vi "Annotate Frame.vi"(6 "Codec":string, 7 "Clip width":i32, 8 "error in (no error)":errorcluster, 9 "Annotation Type":T11, 10 "Annotation":string, 11 "Frame Grabber Data In in":T1={"Camera Session"="", "Frame"=refnum, "AVI Refnum"=refnum, "Codecs"=[], "Frame number"=0, "Tracking File Refnum"=refnum, "Tick Count"=0, "Probe Object"=refnum, "Playback Probe Data"=[], "Rigid Body"={"Position"={"x (mm)"=0.0, "y (mm)"=0.0, "z (mm)"=0.0}, "Orientation"={"Pitch (rad)"=0.0, "Yaw (rad)"=0.0, "Roll (rad)"=0.0}, "Quaternion"={"qx"=0.0, "qy"=0.0, "qz"=0.0, "qw"=0.0}, "Tracked?"=FALSE}, "Total no frames playback"=0, "Video FPS"=0.0, "Camera connected?"=FALSE, "Scene"=refnum, "Cropped Frame"=refnum, "Tracker FPS"=0.0, "Crop ROI"=[], "Presentation Values"=[], "Elapsed time (ms)"=0, "Camera frames playback"=0, "Refnums"={"Live Refnum"=refnum, "Record Refnum"=refnum, "Playback Refnum"=refnum, "Frame Slider Refnum"=refnum, "Pause Refnum"=refnum, "Home Refnum"=refnum, "Set Crop Refnum"=refnum, "Clear Crop Refnum"=refnum, "stop refnum"=refnum, "Playback Rate Refnum"=refnum, "Presentation Refnum"=refnum, "Crop Time Frame Slider Refnum"=refnum, "Cancel Save Refnum"=refnum, "Reverse Playback Refnum"=refnum, "Recording Settings Refnum"=refnum, "Continuous Playback Refnum"=refnum, "Annotation Refnum"=refnum, "Export All Refnum"=refnum, "Export List Refnum"=refnum, "Fill List Refnum"=refnum, "Save Crop Refnum"=refnum, "Skip Forward Refnum"=refnum, "Skip Backward Refnum"=refnum, "Single Annotation Refnum"=refnum, "Load Refnum"=refnum, "Set Start Refnum"=refnum, "Set End Refnum"=refnum, "Add to List Refnum"=refnum, "List of Annotations Refnum"=refnum, "Camera Frame Refnum"=refnum}, "Dimensions"={"Probe Dimensions"={"Probe Width"=0.0, "Probe Depth"=1.0, "Probe Height"=0.0}, "Room Dimensions"={"Room Width"=0.0, "Room Depth"=0.0, "Room Height"=0.0}}, "Playback Data As Strings"=[], "Cropped Tracking File Refnum"=refnum, "Cropped AVI Refnum"=refnum, "Header"=[], "Total euclidian distance"=0.0, "Annotation File Path"=path "", "Playback File Path"=path "", "Size per frame"=0.0, "Ground Truth File Refnum"=refnum, "Annotation Array"=[], "Annotation TIFFs Folder"=path "", "overwriting open file?"=FALSE}) -> (0 "error out":errorcluster, 2 "saving?":bool, 3 "Frame Grabber Data Out":T1={"Camera Session"="", "Frame"=refnum, "AVI Refnum"=refnum, "Codecs"=[], "Frame number"=0, "Tracking File Refnum"=refnum, "Tick Count"=0, "Probe Object"=refnum, "Playback Probe Data"=[], "Rigid Body"={"Position"={"x (mm)"=0.0, "y (mm)"=0.0, "z (mm)"=0.0}, "Orientation"={"Pitch (rad)"=0.0, "Yaw (rad)"=0.0, "Roll (rad)"=0.0}, "Quaternion"={"qx"=0.0, "qy"=0.0, "qz"=0.0, "qw"=0.0}, "Tracked?"=FALSE}, "Total no frames playback"=0, "Video FPS"=0.0, "Camera connected?"=FALSE, "Scene"=refnum, "Cropped Frame"=refnum, "Tracker FPS"=0.0, "Crop ROI"=[], "Presentation Values"=[], "Elapsed time (ms)"=0, "Camera frames playback"=0, "Refnums"={"Live Refnum"=refnum, "Record Refnum"=refnum, "Playback Refnum"=refnum, "Frame Slider Refnum"=refnum, "Pause Refnum"=refnum, "Home Refnum"=refnum, "Set Crop Refnum"=refnum, "Clear Crop Refnum"=refnum, "stop refnum"=refnum, "Playback Rate Refnum"=refnum, "Presentation Refnum"=refnum, "Crop Time Frame Slider Refnum"=refnum, "Cancel Save Refnum"=refnum, "Reverse Playback Refnum"=refnum, "Recording Settings Refnum"=refnum, "Continuous Playback Refnum"=refnum, "Annotation Refnum"=refnum, "Export All Refnum"=refnum, "Export List Refnum"=refnum, "Fill List Refnum"=refnum, "Save Crop Refnum"=refnum, "Skip Forward Refnum"=refnum, "Skip Backward Refnum"=refnum, "Single Annotation Refnum"=refnum, "Load Refnum"=refnum, "Set Start Refnum"=refnum, "Set End Refnum"=refnum, "Add to List Refnum"=refnum, "List of Annotations Refnum"=refnum, "Camera Frame Refnum"=refnum}, "Dimensions"={"Probe Dimensions"={"Probe Width"=0.0, "Probe Depth"=1.0, "Probe Height"=0.0}, "Room Dimensions"={"Room Width"=0.0, "Room Depth"=0.0, "Room Height"=0.0}}, "Playback Data As Strings"=[], "Cropped Tracking File Refnum"=refnum, "Cropped AVI Refnum"=refnum, "Header"=[], "Total euclidian distance"=0.0, "Annotation File Path"=path "", "Playback File Path"=path "", "Size per frame"=0.0, "Ground Truth File Refnum"=refnum, "Annotation Array"=[], "Annotation TIFFs Folder"=path "", "overwriting open file?"=FALSE})   [LabVIEW 2017]
uses:
  Controls/Frame Grabber Data.ctl
  <vilib>/userdefined/High Color/IMAQdx.ctl
  <vilib>/vision/Image Controls.llb/IMAQ Image.ctl
  <vilib>/vision/Avi.llb/IMAQ AVI2 Refnum.ctl
  Controls/Rigid Body Info.ctl
  Controls/Position.ctl
  Controls/Orientation.ctl
  Controls/Refnums.ctl
  Controls/Recording Settings.ctl
  Controls/Operator Settings.ctl
  Controls/Operator.ctl
  Controls/Patient Settings.ctl
  Controls/Dimensions.ctl
  Controls/Room Dimensions.ctl
  Controls/Annotation Type.ctl
  <vilib>/Utility/file.llb/Read Delimited Spreadsheet (string).vi
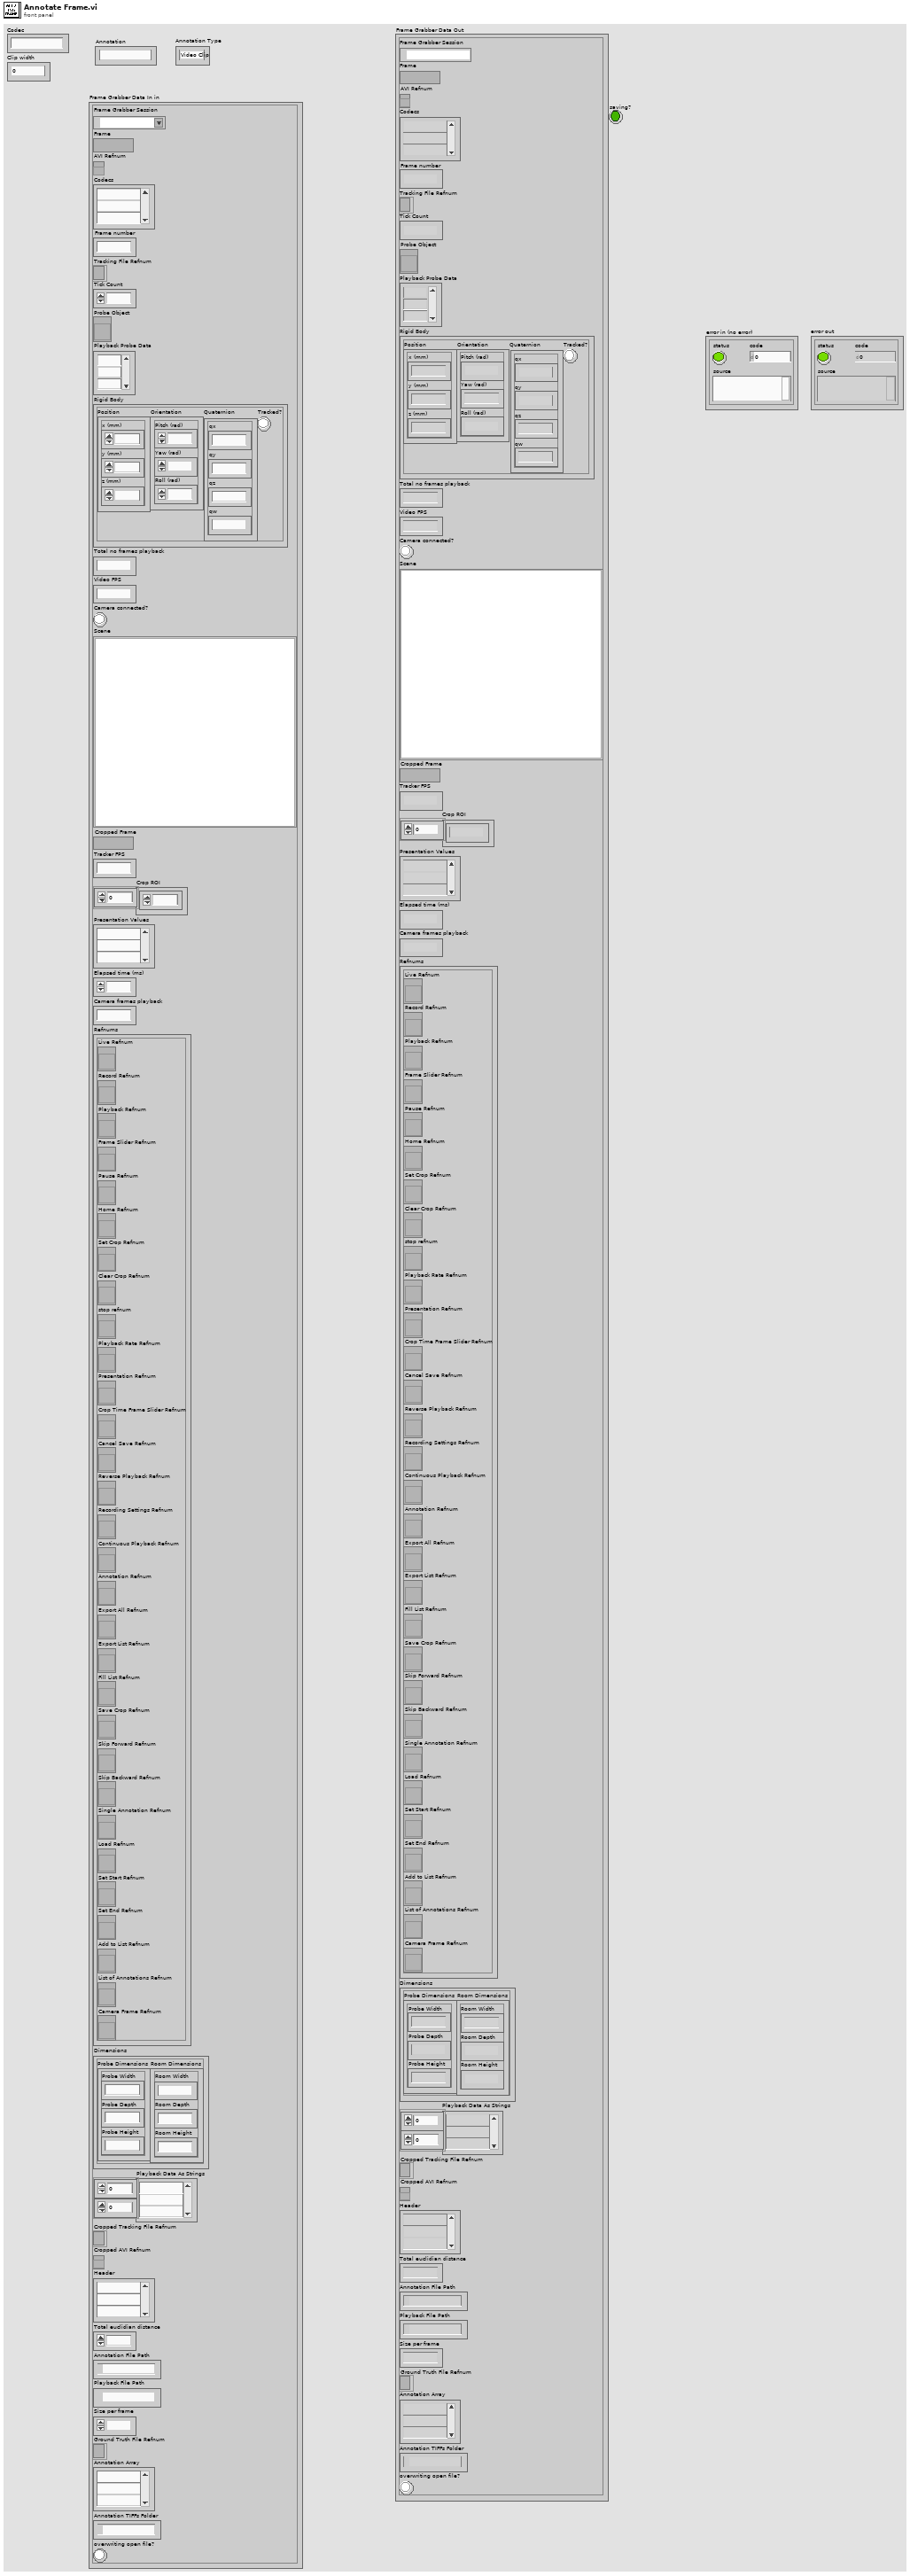
[diagram p1: front panel]
types:
  T1 = typedef "Frame Grabber Data.ctl" = cluster{"Camera Session":T2, "Frame":T3, "AVI Refnum":T4, "Codecs":string[], "Frame number":u32, "Tracking File Refnum":refnum<file>, "Tick Count":u32, "Probe Object":refnum<vi>, "Playback Probe Data":dbl[][], "Rigid Body":T5, "Total no frames playback":i32, "Video FPS":dbl, "Camera connected?":bool, "Scene":refnum<vi>, "Cropped Frame":T3, "Tracker FPS":dbl, "Crop ROI":i32[], "Presentation Values":string[], "Elapsed time (ms)":u32, "Camera frames playback":u32, "Refnums":T8, "Dimensions":T9, "Playback Data As Strings":string[][], "Cropped Tracking File Refnum":refnum<file>, "Cropped AVI Refnum":T4, "Header":string[], "Total euclidian distance":dbl, "Annotation File Path":path, "Playback File Path":path, "Size per frame":dbl, "Ground Truth File Refnum":refnum<file>, "Annotation Array":string[], "Annotation TIFFs Folder":path, "overwriting open file?":bool}
  T2 = typedef "IMAQdx.ctl" = refnum<k21>
  T3 = typedef "IMAQ Image.ctl" = refnum<image>
  T4 = typedef "IMAQ AVI2 Refnum.ctl" = refnum<k20>
  T5 = typedef "Rigid Body Info.ctl" = cluster{"Position":T6, "Orientation":T7, "Quaternion":cluster{"qx":sgl, "qy":sgl, "qz":sgl, "qw":sgl}, "Tracked?":bool}
  T6 = typedef "Position.ctl" = cluster{"x (mm)":sgl, "y (mm)":sgl, "z (mm)":sgl}
  T7 = typedef "Orientation.ctl" = cluster{"Pitch (rad)":sgl, "Yaw (rad)":sgl, "Roll (rad)":sgl}
  T8 = typedef "Refnums.ctl" = cluster{"Live Refnum":refnum<vi>, "Record Refnum":refnum<vi>, "Playback Refnum":refnum<vi>, "Frame Slider Refnum":refnum<vi>, "Pause Refnum":refnum<vi>, "Home Refnum":refnum<vi>, "Set Crop Refnum":refnum<vi>, "Clear Crop Refnum":refnum<vi>, "stop refnum":refnum<vi>, "Playback Rate Refnum":refnum<vi>, "Presentation Refnum":refnum<vi>, "Crop Time Frame Slider Refnum":refnum<vi>, "Cancel Save Refnum":refnum<vi>, "Reverse Playback Refnum":refnum<vi>, "Recording Settings Refnum":refnum<vi>, "Continuous Playback Refnum":refnum<vi>, "Annotation Refnum":refnum<vi>, "Export All Refnum":refnum<vi>, "Export List Refnum":refnum<vi>, "Fill List Refnum":refnum<vi>, "Save Crop Refnum":refnum<vi>, "Skip Forward Refnum":refnum<vi>, "Skip Backward Refnum":refnum<vi>, "Single Annotation Refnum":refnum<vi>, "Load Refnum":refnum<vi>, "Set Start Refnum":refnum<vi>, "Set End Refnum":refnum<vi>, "Add to List Refnum":refnum<vi>, "List of Annotations Refnum":refnum<vi>, "Camera Frame Refnum":refnum<vi>}
  T9 = typedef "Dimensions.ctl" = cluster{"Probe Dimensions":cluster{"Probe Width":sgl, "Probe Depth":sgl, "Probe Height":sgl}, "Room Dimensions":T10}
  T10 = typedef "Room Dimensions.ctl" = cluster{"Room Width":dbl, "Room Depth":dbl, "Room Height":dbl}
  T11 = typedef "Annotation Type.ctl" = enum16{"Video Clip", "Image"}
  T12 = enum16{"open", "replace", "create", "open or create", "replace or create", "replace or create with confirmation"}
  T13 = cluster{"Width":u32, "Height":u32, "Frames Per Second":u32, "Codec":string, "Has Data":bool}
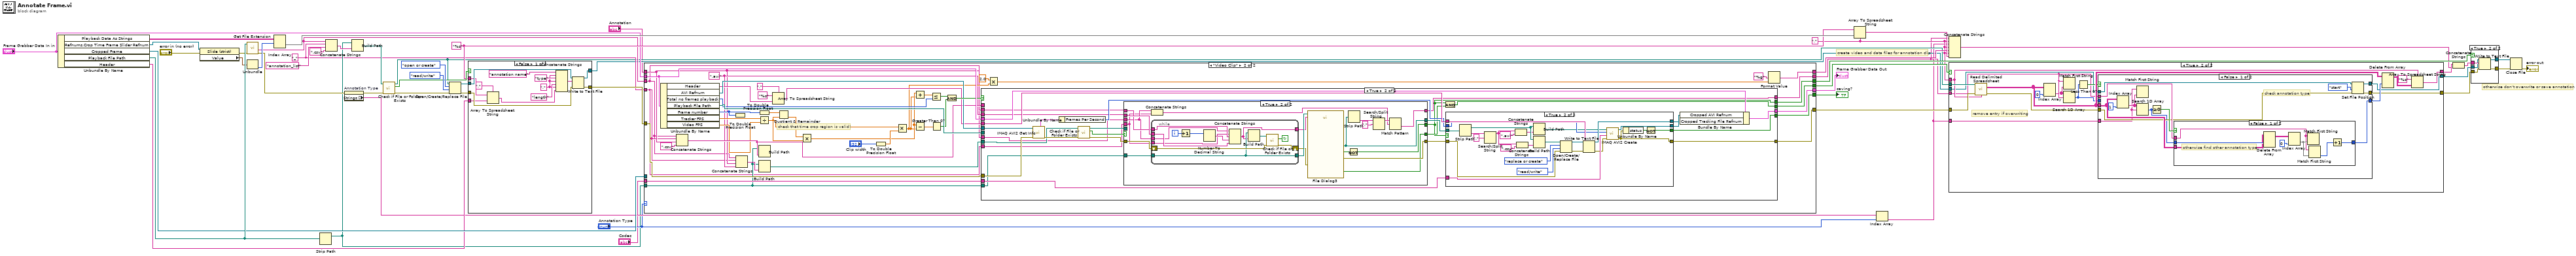
[diagram p0: block diagram]
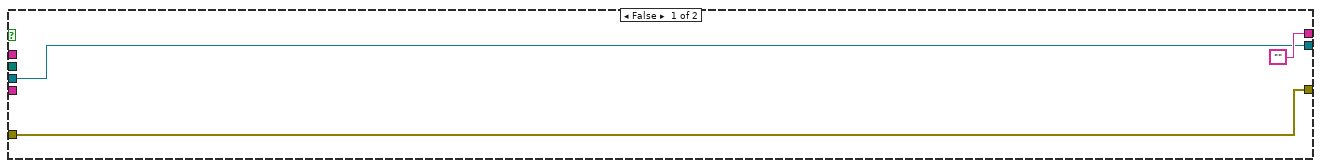
[diagram p2: hidden frame]
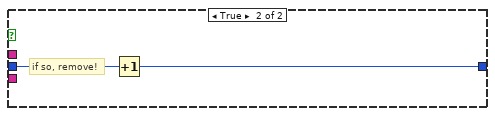
[diagram p3: hidden frame]
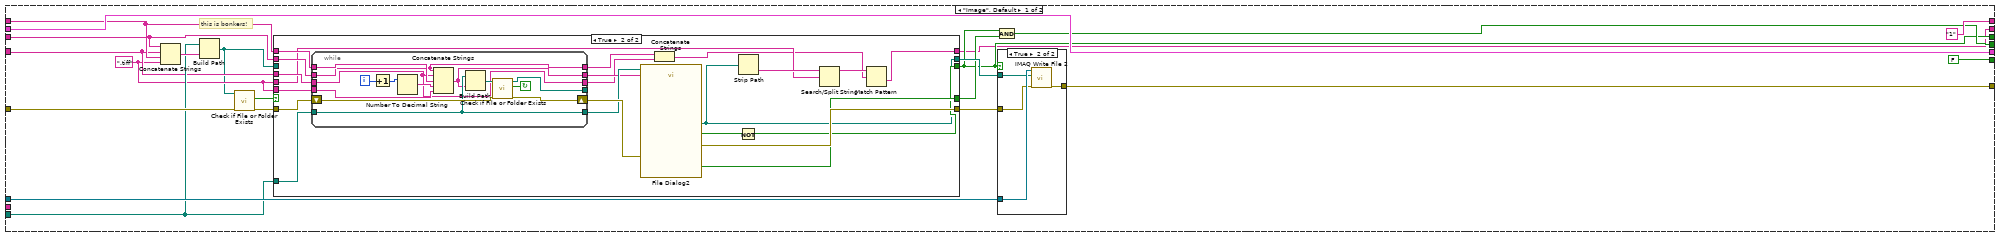
[diagram p6: hidden frame]
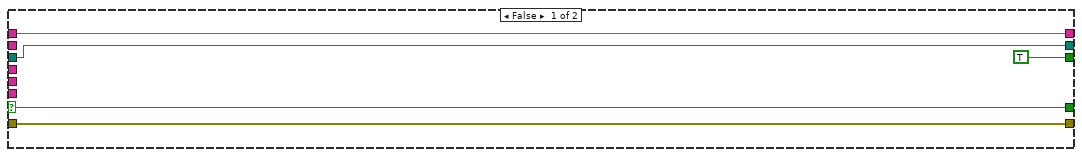
[diagram p7: hidden frame]
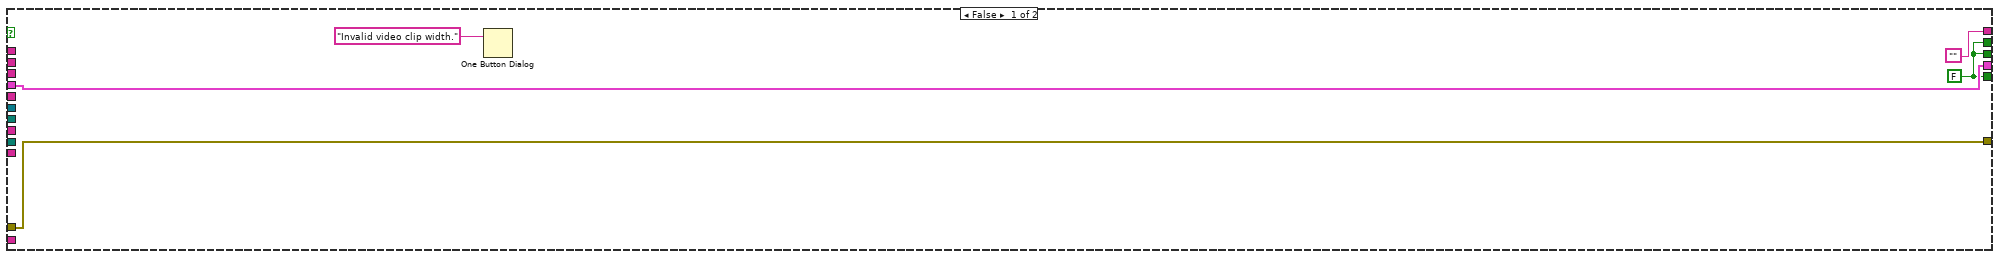
[diagram p9: hidden frame]
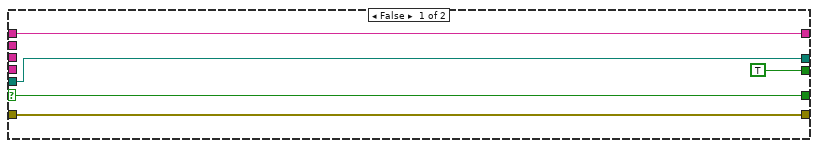
[diagram p10: hidden frame]
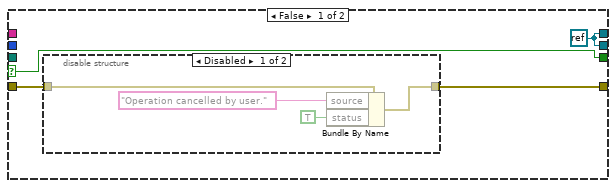
[diagram p11: hidden frame]
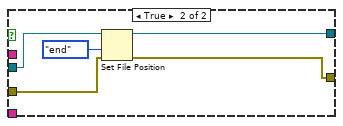
[diagram p13: hidden frame]
diagram:
  w19 = "_" ("string")
  w6 = "," ("delimiter (Tab)")
  w33 = "%s" ("format string")
  # "otherwise don't overwrite or save annotation"
  # "create video and data files for annotation clip"
  n1 = Unbundle By Name("Frame Grabber Data In in") -> ("Playback Data As Strings"=w52:string[][], "Refnums.Crop Time Frame Slider Refnum"=w32:refnum<vi>, "Cropped Frame"=w42:T3, "Playback File Path"=w51:path, "Header"=w39:string[])
  n2 = property class="Slide (strict)"(reference=w32, error in="error in (no error)") -> (error out=w28:errorcluster, "Value"=w31:cluster{i32, i32, i32})  [unwired: 1 out]
  n3 = call <vilib>:"Get File Extension.vi"("error in (no error)"=w28, "file"=w51) -> ("error out"=w27:errorcluster, "filename without extension"=w20:string)  [unwired: 5 in, 3 out]
  n4 = Unbundle(w31) -> (w30:i32)  [unwired: 2 out]
  n5 = Index Array(array=w52, index (row)=w30) -> (element=w34:string[])  [unwired: 1 in]
  n6 = Strip Path(path=w51) -> (stripped path=w21:path)  [unwired: 1 out]
  n7 = Concatenate Strings(w20, w19, "annotation_list" ("string"), ".csv" ("string")) -> (w50:string)
  n8 = property on="Annotation Type" class="Enum (strict)"(error in=w27) -> (error out=w26:errorcluster, "Strings []"=w25:string[])  [unwired: 1 in, 1 out]
  n9 = Build Path(base path=w21, name or relative path=w50) -> (appended path=w41:path)
  n10 = call <vilib>:"Check if File or Folder Exists.vi"("error in (no error)"=w26, "path"=w41) -> ("error out"=w40:errorcluster, "file or folder exists?"=w37:bool, "dup path"=w12:path)  [unwired: 7 in]
  n11 = Open/Create/Replace File(file path (use dialog)=w12, error in=w40, operation (0:open)=T12."open or create", access (0:read/write)=enum16{"read/write", "read-only", "write-only"}."read/write") -> (refnum out=w35:refnum<file>, error out=w38:errorcluster)  [unwired: 2 in, 1 out]
  n12 = case shown="False" w37 {
    tunnel: w39 -> [w59 _]
    tunnel: w38 -> [w64 w70]
    tunnel: [w63 w67] -> w36
    tunnel: w35 -> [w62 w69]
    tunnel: [w61 w68] -> w4
    tunnel: w33 -> [w56 _]
    frame False {
      w53 = "," ("string")
      n13 = Array To Spreadsheet String(delimiter (Tab)=",", array=w59, 3:w56) -> (spreadsheet string=w57:string)
      n14 = Concatenate Strings("annotation name" ("string"), w53, "type" ("string"), w53, "length" ("string"), w53, w57) -> (w60:string)
      n15 = Write to Text File(file (use dialog)=w62, text=w60, error in=w64) -> (refnum out=w61:refnum<file>, error out=w63:errorcluster)  [unwired: 1 in, 1 out]
    }
    frame True {
      n16 = Set File Position(refnum=w69, from (0:start)=enum16{"start", "end", "current"}."end", error in=w70) -> (refnum out=w68:refnum<file>, error out=w67:errorcluster)  [unwired: 1 in]
    }
  }
  n17 = case shown="\"Video Clip\"" "Annotation Type" {
    tunnel: [w91 w178] -> w11
    tunnel: w42 -> [w90 _]
    tunnel: w36 -> [w85 w179]
    tunnel: [w89 w176] -> w23
    tunnel: "Frame Grabber Data In in" -> [w89 w177]
    tunnel: w21 -> [w80 w142]
    tunnel: w20 -> [w78 w138]
    tunnel: w19 -> [w79 w139]
    tunnel: "Annotation" -> [w81 w140]
    tunnel: "Codec" -> [_ w175]
    tunnel: [FALSE ("status") w159] -> w17
    tunnel: ["1" ("output string") w145] -> w15
    tunnel: [w74 w144] -> w14
    tunnel: [w86 w143] -> w13
    tunnel: [w72 w137] -> w2
    frame "Image", Default {
      w73 = ".tiff" ("string")
      # "this is bonkers!"
      n18 = Concatenate Strings(w78, w79, w81, w73) -> (w84:string)
      n19 = Build Path(base path=w80, name or relative path=w84) -> (appended path=w71:path)
      n20 = call <vilib>:"Check if File or Folder Exists.vi"("error in (no error)"=w85, "path"=w71) -> ("error out"=w82:errorcluster, "file or folder exists?"=w83:bool)  [unwired: 7 in, 1 out]
      n21 = case shown="True" w83 {
        selector: w83 -> [w94 _]
        tunnel: w82 -> [w96 w117]
        tunnel: [w96 w115] -> w77
        tunnel: w80 -> [_ w110]
        tunnel: [w92 w104] -> w76
        tunnel: [TRUE w112] -> w74
        tunnel: [w94 w114] -> w75
        tunnel: w81 -> [w93 w111]
        tunnel: w73 -> [_ w109]
        tunnel: w79 -> [_ w108]
        tunnel: w78 -> [_ w107]
        tunnel: w73 -> [_ w102]
        tunnel: [w93 w97] -> w72
        tunnel: w71 -> [w92 _]
        frame False {
        }
        frame True {
          n22 = while {
            shift-right: [w130] -> w116
            shift-left: w117 -> [w123]
            tunnel: [w129] -> _
            tunnel: w111 -> [w125]
            tunnel: w110 -> [w121]
            tunnel: w109 -> [w124]
            tunnel: w108 -> [w119]
            tunnel: w107 -> [w118]
            tunnel: [w121] -> w106
            tunnel: [w120] -> w105
            tunnel: [w119] -> w100
            tunnel: [w118] -> w99
            i -> [w128]
            stop <- w131 continue-if-true
            n23 = Increment(x=w128) -> (x+1=w127:i32)
            n24 = Number To Decimal String(number=w127) -> (decimal integer string=w126:string)  [unwired: 1 in]
            n25 = Concatenate Strings(w118, w119, w125, w126, w124) -> (w120:string)
            n26 = Build Path(base path=w121, name or relative path=w120) -> (appended path=w122:path)
            n27 = call <vilib>:"Check if File or Folder Exists.vi"("error in (no error)"=w123, "path"=w122) -> ("error out"=w130:errorcluster, "file or folder exists?"=w131:bool, "dup path"=w129:path)  [unwired: 7 in]
          }
          n28 = call "File Dialog2"("start path"=w106, "default name"=w105, "error in"=w116) -> ("selected path"=w104:path, "exists"=w114:bool, "cancelled"=w113:bool, "error out"=w115:errorcluster)  [unwired: 9 in]
          n29 = Concatenate Strings(w99, w100) -> (w98:string)
          n30 = Not(x=w113) -> (.not. x?=w112:bool)
          n31 = Strip Path(path=w104) -> (name=w103:string)  [unwired: 1 out]
          n32 = Search/Split String(string=w103, search string/char (-)=w102) -> (substring before match=w101:string)  [unwired: 1 in, 2 out]
          n33 = Match Pattern(string=w101, regular expression=w98) -> (after substring=w97:string)  [unwired: 1 in, 3 out]
        }
      }
      n34 = And(x=w74, y=w75) -> (x .and. y?=w86:bool)
      n35 = case shown="True" w74 {
        tunnel: [w132 w133] -> w91
        tunnel: w90 -> [_ w136]
        tunnel: w77 -> [w132 w135]
        tunnel: w76 -> [_ w134]
        frame False {
        }
        frame True {
          n36 = call-poly "IMAQ Write File 2"("error in (no error)"=w135, "File Path"=w134, "Image"=w136) -> ("error out"=w133:errorcluster)  [unwired: 7 in, 1 out]
        }
      }
    }
    frame "Video Clip" {
      w141 = ".avi" ("string")
      # "check that time crop region is valid!"
      n37 = Unbundle By Name(w177) -> ("Header"=w170:string[], "AVI Refnum"=w171:T4, "Total no frames playback"=w161:i32, "Playback File Path"=w174:path, "Frame number"=w154:u32, "Tracker FPS"=w158:dbl, "Video FPS"=w157:dbl)
      n38 = Concatenate Strings(w138, w139, w140, ".csv" ("string")) -> (w164:string)
      n39 = To Double Precision Float(number=w154) -> ()  [unwired: 1 out]
      n40 = Concatenate Strings(w138, w139, w140, w141) -> (w180:string)
      n41 = To Double Precision Float(number=w154) -> (double precision float=w152:dbl)
      n42 = Divide(x=w158, y=w157) -> (x/y=w150:dbl)
      n43 = Build Path(base path=w142, name or relative path=w164) -> ()  [unwired: 1 out]
      n44 = Build Path(base path=w142, name or relative path=w180) -> (appended path=w166:path)
      n45 = Array To Spreadsheet String(delimiter (Tab)=",", array=w170, 3:"%s" ("format string")) -> (spreadsheet string=w167:string)
      n46 = Quotient & Remainder(x=w152, y=w150) -> (floor(x/y)=w153:dbl)  [unwired: 1 out]
      n47 = Multiply(x=w153, y=w150) -> (x*y=w151:dbl)
      n48 = To Double Precision Float(number="Clip width") -> (double precision float=w156:dbl)
      n49 = Multiply(x=w150, y=w156) -> (x*y=w149:dbl)
      n50 = Add(x=w151, y=w149) -> (x+y=w162:dbl)
      n51 = Subtract(x=w151, y=w149) -> (x-y=w163:dbl)
      n52 = Less Or Equal?(x=w162, y=w161) -> (x <= y?=w160:bool)
      n53 = Greater Than 0?(x=w163) -> (x > 0?=w172:bool)
      n54 = And(x=w160, y=w172) -> (x .and. y?=w173:bool)
      n55 = case shown="True" w173 {
        tunnel: w167 -> [_ w213]
        tunnel: w177 -> [w185 w212]
        tunnel: [w185 w210] -> w176
        tunnel: w171 -> [_ w208]
        tunnel: w179 -> [w184 w205]
        tunnel: w174 -> [_ _]
        tunnel: [w182 w200] -> w159
        tunnel: w175 -> [_ w204]
        tunnel: [w184 w203] -> w178
        tunnel: w166 -> [_ w201]
        tunnel: w164 -> [_ _]
        tunnel: [w182 w191] -> w144
        tunnel: [w182 w194] -> w143
        tunnel: w142 -> [_ w198]
        tunnel: w141 -> [_ w190]
        tunnel: w140 -> [_ w189]
        tunnel: w139 -> [_ w188]
        tunnel: w138 -> [_ w187]
        tunnel: ["" w186] -> w137
        frame False {
          w182 = FALSE ("status")
          n56 = One Button Dialog(message="Invalid video clip width.") -> ()  [unwired: 1 in, 1 out]
        }
        frame True {
          n57 = call "IMAQ AVI2 Get Info"("error in (no error)"=w205, "AVI Refnum"=w208) -> ("error out"=w202:errorcluster, "Frame Data"=w207:T13)  [unwired: 5 in, 3 out]
          n58 = Unbundle By Name(w207) -> ("Frames Per Second"=w206:u32)
          n59 = call <vilib>:"Check if File or Folder Exists.vi"("error in (no error)"=w202, "path"=w201) -> ("error out"=w199:errorcluster, "file or folder exists?"=w193:bool, "dup path"=w195:path)  [unwired: 7 in]
          n60 = case shown="True" w193 {
            selector: w193 -> [w215 _]
            tunnel: w199 -> [w218 w237]
            tunnel: w198 -> [_ w236]
            tunnel: [w218 w232] -> w197
            tunnel: [w217 w226] -> w196
            tunnel: w195 -> [w217 _]
            tunnel: [w215 w230] -> w192
            tunnel: [TRUE w229] -> w191
            tunnel: w190 -> [_ w228]
            tunnel: w189 -> [w214 w227]
            tunnel: w188 -> [_ w219]
            tunnel: w187 -> [_ w220]
            tunnel: [w214 w225] -> w186
            frame False {
            }
            frame True {
              n61 = Concatenate Strings(w220, w219) -> (w221:string)
              n62 = while {
                shift-right: [w248] -> w233
                shift-left: w237 -> [w249]
                tunnel: w236 -> [w247]
                tunnel: [w247] -> w235
                tunnel: [w242] -> w234
                tunnel: w228 -> [w241]
                tunnel: w227 -> [w240]
                tunnel: w219 -> [w239]
                tunnel: w220 -> [w238]
                i -> [w245]
                stop <- w250 continue-if-true
                n63 = Increment(x=w245) -> (x+1=w246:i32)
                n64 = Number To Decimal String(number=w246) -> (decimal integer string=w244:string)  [unwired: 1 in]
                n65 = Concatenate Strings(w238, w239, w240, w244, w241) -> (w242:string)
                n66 = Build Path(base path=w247, name or relative path=w242) -> (appended path=w243:path)
                n67 = call <vilib>:"Check if File or Folder Exists.vi"("error in (no error)"=w249, "path"=w243) -> ("error out"=w248:errorcluster, "file or folder exists?"=w250:bool)  [unwired: 7 in, 1 out]
              }
              n68 = call "File Dialog3"("start path"=w235, "default name"=w234, "error in"=w233) -> ("selected path"=w226:path, "exists"=w230:bool, "cancelled"=w231:bool, "error out"=w232:errorcluster)  [unwired: 9 in]
              n69 = Not(x=w231) -> (.not. x?=w229:bool)
              n70 = Strip Path(path=w226) -> (name=w224:string)  [unwired: 1 out]
              n71 = Search/Split String(string=w224, search string/char (-)=".") -> (substring before match=w222:string)  [unwired: 1 in, 2 out]
              n72 = Match Pattern(string=w222, regular expression=w221) -> (after substring=w225:string)  [unwired: 1 in, 3 out]
            }
          }
          n73 = And(x=w191, y=w192) -> (x .and. y?=w194:bool)
          n74 = case shown="True" w191 {
            selector: w191 -> [w251 _]
            tunnel: w213 -> [_ w284]
            tunnel: [w254 w283] -> w211
            tunnel: [w254 w282] -> w209
            tunnel: w204 -> [_ w281]
            tunnel: w206 -> [_ w280]
            tunnel: [w253 w278] -> w203
            tunnel: w197 -> [w252 w277]
            tunnel: w196 -> [_ w270]
            tunnel: [w251 w271] -> w200
            frame False {
              w254 = refnum<k0> refnum
              n75 = disable-structure shown="Disabled" {
                disable-tunnel: [w258 w259] -> w253
                disable-tunnel: w252 -> [w255 w259]
                frame Disabled {
                  n76 = Bundle By Name(cluster=w255, "source"="Operation cancelled by user.", "status"=TRUE) -> (w258:errorcluster)
                }
                frame Enabled {
                }
              }
            }
            frame True {
              n77 = Strip Path(path=w270) -> (stripped path=w264:path, name=w268:string)
              n78 = Search/Split String(string=w268, search string/char (-)=".") -> (substring before match=w267:string)  [unwired: 1 in, 2 out]
              n79 = Concatenate Strings(w267, ".avi" ("string")) -> (w263:string)
              n80 = Concatenate Strings(w267, ".csv" ("string")) -> (w261:string)
              n81 = Build Path(base path=w264, name or relative path=w263) -> (appended path=w262:path)
              n82 = Build Path(base path=w264, name or relative path=w261) -> (appended path=w260:path)
              n83 = Open/Create/Replace File(file path (use dialog)=w260, error in=w277, operation (0:open)=T12."replace or create", access (0:read/write)=enum16{"read/write", "read-only", "write-only"}."read/write") -> (refnum out=w273:refnum<file>, error out=w274:errorcluster)  [unwired: 2 in, 1 out]
              n84 = Write to Text File(file (use dialog)=w273, text=w284, error in=w274) -> (refnum out=w282:refnum<file>, error out=w279:errorcluster)  [unwired: 1 in, 1 out]
              n85 = call "IMAQ AVI2 Create"("error in (no error)"=w279, "Codec"=w281, "Frames Per Second"=w280, "AVI Path"=w262) -> ("error out"=w278:errorcluster, "AVI Refnum"=w283:T4)  [unwired: 6 in]
              n86 = Unbundle By Name(w278) -> ("status"=w272:bool)
              n87 = Not(x=w272) -> (.not. x?=w271:bool)
            }
          }
          n88 = Bundle By Name(cluster=w212, "Cropped AVI Refnum"=w211, "Cropped Tracking File Refnum"=w209) -> (w210:T1)
        }
      }
      n89 = Multiply(x=2.0, y=w149) -> (x*y=w147:dbl)
      n90 = Format Value(format string="%g", value (0)=w147) -> (output string=w145:string)  [unwired: 1 in]
    }
  }
  "Frame Grabber Data Out" <- w23
  "saving?" <- w17
  n91 = Array To Spreadsheet String(delimiter (Tab)=w6, array=w34, 3:w33) -> (spreadsheet string=w16:string)
  n92 = Index Array(array=w25, index="Annotation Type") -> (element=w5:string)
  n93 = Concatenate Strings(w2, w6, w5, w6, w15, w6, w16) -> (w9:string)
  n94 = case shown="True" w13 {
    tunnel: w12 -> [_ w305]
    tunnel: w11 -> [w287 w304]
    tunnel: w2 -> [_ w290]
    tunnel: ["" w301] -> w10
    tunnel: [w287 w291] -> w7
    tunnel: w6 -> [_ w299]
    tunnel: w5 -> [_ w297]
    tunnel: w4 -> [w285 w293]
    tunnel: [w285 w292] -> w3
    frame False {
    }
    frame True {
      # "remove entry if overwriting"
      n95 = call-poly <vilib>:"Read Delimited Spreadsheet.vi"("file path (dialog if empty)"=w305, "error in (no error)"=w304, "delimiter (\\t)"=w299) -> ("all rows"=w298:string[][], "error out"=w294:errorcluster)  [unwired: 7 in, 4 out]
      n96 = Index Array(array=w298, index (col)=0 ("disabled index (col)")) -> (element=w289:string[])  [unwired: 1 in]
      n97 = Match First String(2:w289, 3:w290) -> ()  [unwired: 2 out]
      n98 = Search 1D Array(1D array=w289, element=w290) -> (index of element=w288:i32)  [unwired: 1 in]
      n99 = Less Than 0?(x=w288) -> (x < 0?=w295:bool)
      n100 = case shown="False" w295 {
        tunnel: w298 -> [w315 _]
        tunnel: w297 -> [w307 _]
        tunnel: [w316 w331] -> w296
        tunnel: w288 -> [_ w331]
        tunnel: w290 -> [w314 _]
        tunnel: w294 -> [w313 w329]
        tunnel: w293 -> [w312 w330]
        tunnel: [w311 w330] -> w292
        tunnel: [w310 w329] -> w291
        frame False {
          # "check annotation type"
          n101 = Index Array(array=w315, index (col)=1 ("disabled index (col)")) -> (element=w308:string[])  [unwired: 1 in]
          n102 = Match First String(2:w308, 3:w307) -> ()  [unwired: 2 out]
          n103 = Search 1D Array(1D array=w308, element=w307) -> (index of element=w306:i32)  [unwired: 1 in]
          n104 = Greater Or Equal To 0?(x=w306) -> (x >= 0?=w317:bool)
          n105 = case shown="False" w317 {
            tunnel: w306 -> [w326 w328]
            tunnel: [w322 w327] -> w316
            tunnel: w315 -> [w325 _]
            tunnel: w314 -> [w320 _]
            frame False {
              # "otherwise find other annotation type"
              n106 = Delete From Array(array=w325, index (row)=w326) -> (array with subset deleted=w324:string[][])  [unwired: 2 in, 1 out]
              n107 = Index Array(array=w324, index (col)=0 ("disabled index (col)")) -> (element=w321:string[])  [unwired: 1 in]
              n108 = Match First String(2:w321, 3:w320) -> ()  [unwired: 2 out]
              n109 = Match First String(2:w321, 3:w320) -> (0:w319:i32)  [unwired: 1 out]
              n110 = Increment(x=w319) -> (x+1=w322:i32)
            }
            frame True {
              # "if so, remove!"
              n111 = Increment(x=w328) -> (x+1=w327:i32)
            }
          }
          n112 = Set File Position(refnum=w312, from (0:start)=enum16{"start", "end", "current"}."start", error in=w313) -> (refnum out=w311:refnum<file>, error out=w310:errorcluster)  [unwired: 1 in]
        }
        frame True {
        }
      }
      n113 = Delete From Array(array=w298, index (row)=w296) -> (array with subset deleted=w302:string[][])  [unwired: 2 in, 1 out]
      n114 = Array To Spreadsheet String(delimiter (Tab)=w299, array=w302, 3:"%s" ("format string")) -> (spreadsheet string=w301:string)
    }
  }
  n115 = Concatenate Strings(w10, w9) -> (w8:string)
  n116 = case shown="True" w14 {
    tunnel: w7 -> [w333 w338]
    tunnel: w8 -> [_ w337]
    tunnel: [w333 w336] -> w47
    tunnel: [w332 w335] -> w46
    tunnel: w3 -> [w332 w334]
    frame False {
    }
    frame True {
      n117 = Write to Text File(file (use dialog)=w334, text=w337, error in=w338) -> (refnum out=w335:refnum<file>, error out=w336:errorcluster)  [unwired: 1 in, 1 out]
    }
  }
  n118 = Close File(refnum=w46, error in=w47) -> (error out=→"error out":errorcluster)  [unwired: 1 out]
